vi "AddChangeInWindow(SubVI).vi"(6 "CmbBox Refnum":refnum<vi>, 7 "Add/Change":enum16{"Add", "Change"}(ring), 8 "Error In":errorcluster, 9 "Arr Refnum":refnum<vi>, 10 "Clust Refnum":refnum<vi>, 11 "Digital in":refnum<vi>) -> (0 "Error Out":errorcluster)   [LabVIEW 2018]
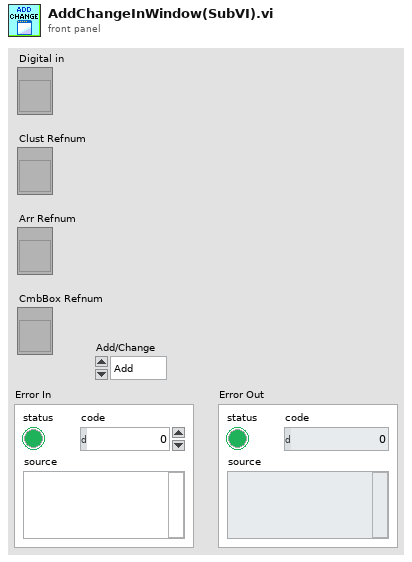
[diagram p1: front panel]
types:
  T1 = typedef "Line.ctl" = cluster{"Width":dbl, "Color":i64, "Array Oy":dbl[], "Array Ox":dbl[], "Name":string, "Plot Visible":T2}
  T2 = typedef "View.ctl" = bool
  T3 = typedef "LVComboBoxStrsAndValuesArrayTypeDef.ctl" = cluster{"String":string, "Value":string}[]
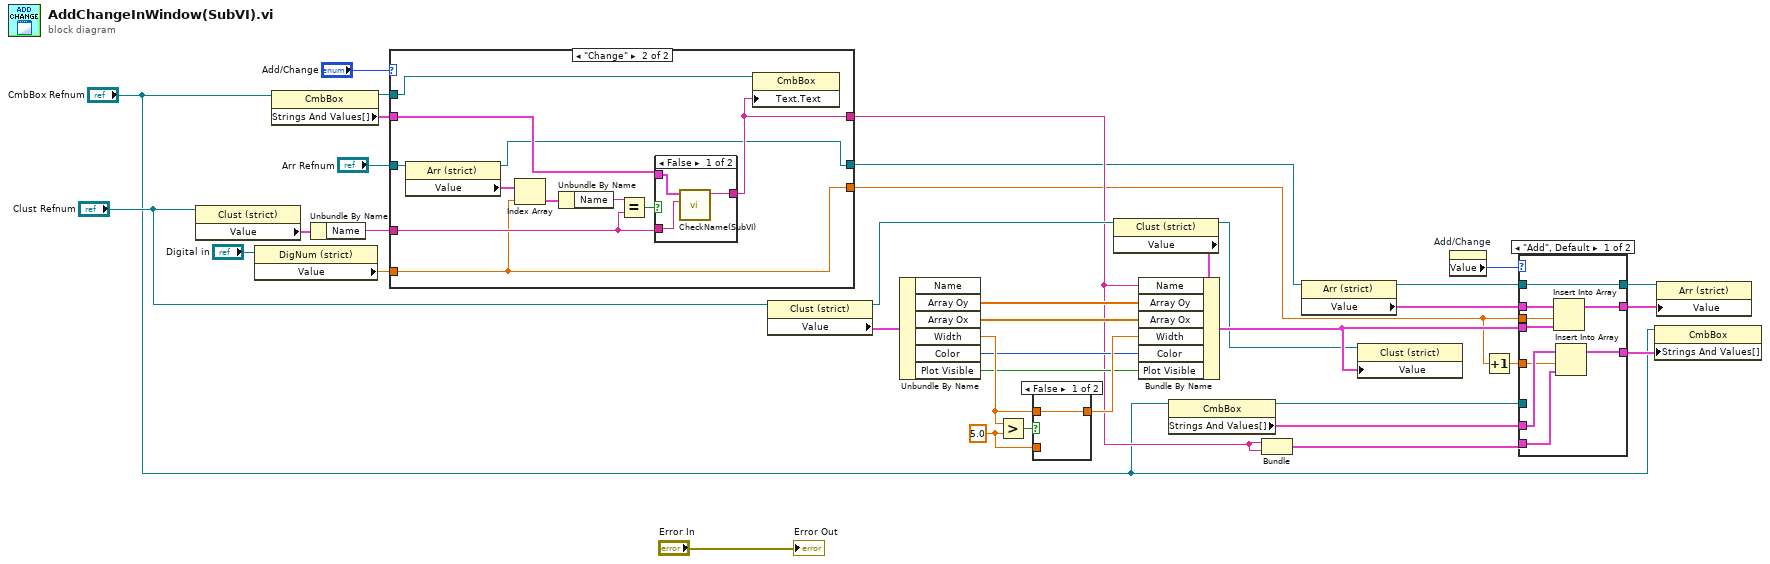
[diagram p0: block diagram]
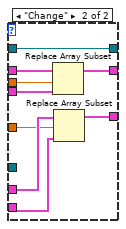
[diagram p2: hidden frame]
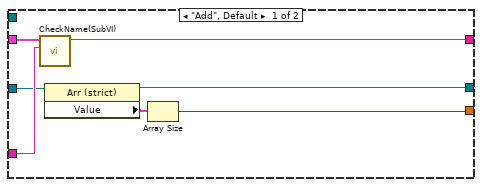
[diagram p4: hidden frame]
diagram:
  w24 = 5.0 ("y")
  n1 = property on="Property Node" class="Clust (strict)"(reference="Clust Refnum") -> ("Value"=w35:T1)  [unwired: 1 in, 2 out]
  n2 = property on="Property Node" class="DigNum (strict)"(reference="Digital in") -> ("Value"=w29:dbl)  [unwired: 1 in, 2 out]
  n3 = property on="Property Node" class="CmbBox"(reference="CmbBox Refnum") -> (reference out=w31:refnum<vi>, "Strings And Values[]"=w33:T3)  [unwired: 1 in, 1 out]
  n4 = Unbundle By Name(w35) -> ("Name"=w34:string)
  n5 = case shown="\"Change\"" "Add/Change" {
    tunnel: w34 -> [w43 w51]
    tunnel: w33 -> [w44 w50]
    tunnel: "Arr Refnum" -> [w42 w49]
    tunnel: w31 -> [_ w46]
    tunnel: [w40 w45] -> w3
    tunnel: w29 -> [_ w45]
    tunnel: [w39 w48] -> w12
    tunnel: [w38 w47] -> w11
    frame "Add", Default {
      n6 = call "CheckName(SubVI).vi"("Name In"=w43, "Strings And Values[]"=w44) -> ("Name Out"=w39:string)  [unwired: 8 in, 1 out]
      n7 = property on="Property Node" class="Arr (strict)"(reference=w42) -> (reference out=w38:refnum<vi>, "Value"=w41:T1[])  [unwired: 1 in, 1 out]
      n8 = Array Size(array=w41) -> (size(s)=w40:i32)
    }
    frame "Change" {
      n9 = property on="Property Node" class="Arr (strict)"(reference=w49) -> (reference out=w47:refnum<vi>, "Value"=w52:T1[])  [unwired: 1 in, 1 out]
      n10 = Index Array(array=w52, index=w45) -> (element=w53:T1)
      n11 = Unbundle By Name(w53) -> ("Name"=w55:string)
      n12 = Equal?(x=w55, y=w51) -> (x = y?=w54:bool)
      n13 = case shown="False" w54 {
        tunnel: w51 -> [w58 w59]
        tunnel: w50 -> [w57 _]
        tunnel: [w56 w59] -> w48
        frame False {
          n14 = call "CheckName(SubVI).vi"("Name In"=w58, "Strings And Values[]"=w57) -> ("Name Out"=w56:string)  [unwired: 8 in, 1 out]
        }
        frame True {
        }
      }
      n15 = property on="Property Node" class="CmbBox"(reference=w46, "Text.Text"=w48) -> ()  [unwired: 1 in, 2 out]
    }
  }
  n16 = property on="Property Node" class="Clust (strict)"(reference="Clust Refnum") -> (reference out=w13:refnum<vi>, "Value"=w14:T1)  [unwired: 1 in, 1 out]
  n17 = Unbundle By Name(w14) -> ("Array Oy"=w17:dbl[], "Array Ox"=w18:dbl[], "Width"=w25:dbl, "Color"=w20:i64, "Plot Visible"=w19:T2)  [unwired: 1 out]
  n18 = Greater?(x=w25, y=w24) -> (0:w23:bool)
  n19 = case shown="False" w23 {
    tunnel: w24 -> [_ w61]
    tunnel: w25 -> [w60 _]
    tunnel: [w60 w61] -> w26
    frame False {
    }
    frame True {
    }
  }
  n20 = property on="Property Node" class="Clust (strict)"(reference=w13) -> (reference out=w10:refnum<vi>, "Value"=w16:T1)  [unwired: 1 in, 1 out]
  n21 = Bundle By Name(cluster=w16, "Name"=w12, "Array Oy"=w17, "Array Ox"=w18, "Width"=w26, "Color"=w20, "Plot Visible"=w19) -> (w27:T1)
  n22 = property on="Property Node" class="CmbBox"(reference="CmbBox Refnum") -> (reference out=w8:refnum<vi>, "Strings And Values[]"=w28:T3)  [unwired: 1 in, 1 out]
  n23 = Bundle("Name"=w12, "Name"=w12) -> (w22:cluster{"Name":string, "Name":string})  [unwired: 1 in]
  n24 = property on="Property Node" class="Arr (strict)"(reference=w11) -> (reference out=w9:refnum<vi>, "Value"=w21:T1[])  [unwired: 1 in, 1 out]
  n25 = property on="Property Node" class="Clust (strict)"(reference=w10, "Value"=w27) -> ()  [unwired: 1 in, 2 out]
  n26 = property on="Add/Change" class="Enum (strict)"() -> ("Value"=w1:enum16{"Add", "Change"})  [unwired: 2 in, 2 out]
  n27 = Increment(x=w3) -> (x+1=w2:dbl)
  n28 = case shown="\"Add\", Default" w1 {
    tunnel: w28 -> [w66 w79]
    tunnel: w27 -> [w68 w78]
    tunnel: w22 -> [w64 w77]
    tunnel: w21 -> [w69 w76]
    tunnel: w3 -> [w70 w75]
    tunnel: w9 -> [w62 w72]
    tunnel: w8 -> [_ _]
    tunnel: [w67 w74] -> w7
    tunnel: [w63 w73] -> w6
    tunnel: [w62 w72] -> w5
    tunnel: w2 -> [w65 w71]
    frame "Add", Default {
      n29 = Insert Into Array(array=w69, index=w70, new element=w68) -> (w67:T1[])
      n30 = Insert Into Array(array=w66, index=w65, new element=w64) -> (w63:T3)
    }
    frame "Change" {
      n31 = Replace Array Subset(array=w76, new element=w78, index=w75) -> (w74:T1[])
      n32 = Replace Array Subset(array=w79, new element=w77, index=w71) -> (w73:T3)
    }
  }
  n33 = property on="Property Node" class="CmbBox"(reference="CmbBox Refnum", "Strings And Values[]"=w6) -> ()  [unwired: 1 in, 2 out]
  n34 = property on="Property Node" class="Arr (strict)"(reference=w5, "Value"=w7) -> ()  [unwired: 1 in, 2 out]
  "Error Out" <- "Error In"
